vi "Controller - State Entry.vi"(8 "error in (no error)":errorcluster, 11 "View Model":T1) -> (0 "error out":errorcluster, 3 "View Model":T1)   [LabVIEW 2017]
doc: "Realized initial transition between current and next controller's states."
uses:
  Model/Controls/View Model.ctl
  Model/Controls/Shared Model.ctl
  Error Handler/Controls/Error Model.ctl
  Error Handler/Controls/Error Message.ctl
  Error Handler/Controls/Error Type.ctl
  Configuration/Controls/Config Model.ctl
  Configuration/Controls/Config DB Message.ctl
  Configuration/Controls/Config DB Command.ctl
  Configuration/Controls/Config DB Overhead.ctl
  Configuration/Controls/Config DB Record1.ctl
  Configuration/Controls/Config DB Record2.ctl
  Controls/Controller Wash Step.ctl
  Views/Vehicle Position Simulation View/Controls/Vehicle - Position.ctl
  Controls/Controller Model.ctl
  Controls/Controller Overhead.ctl
  Controls/Controller State.ctl
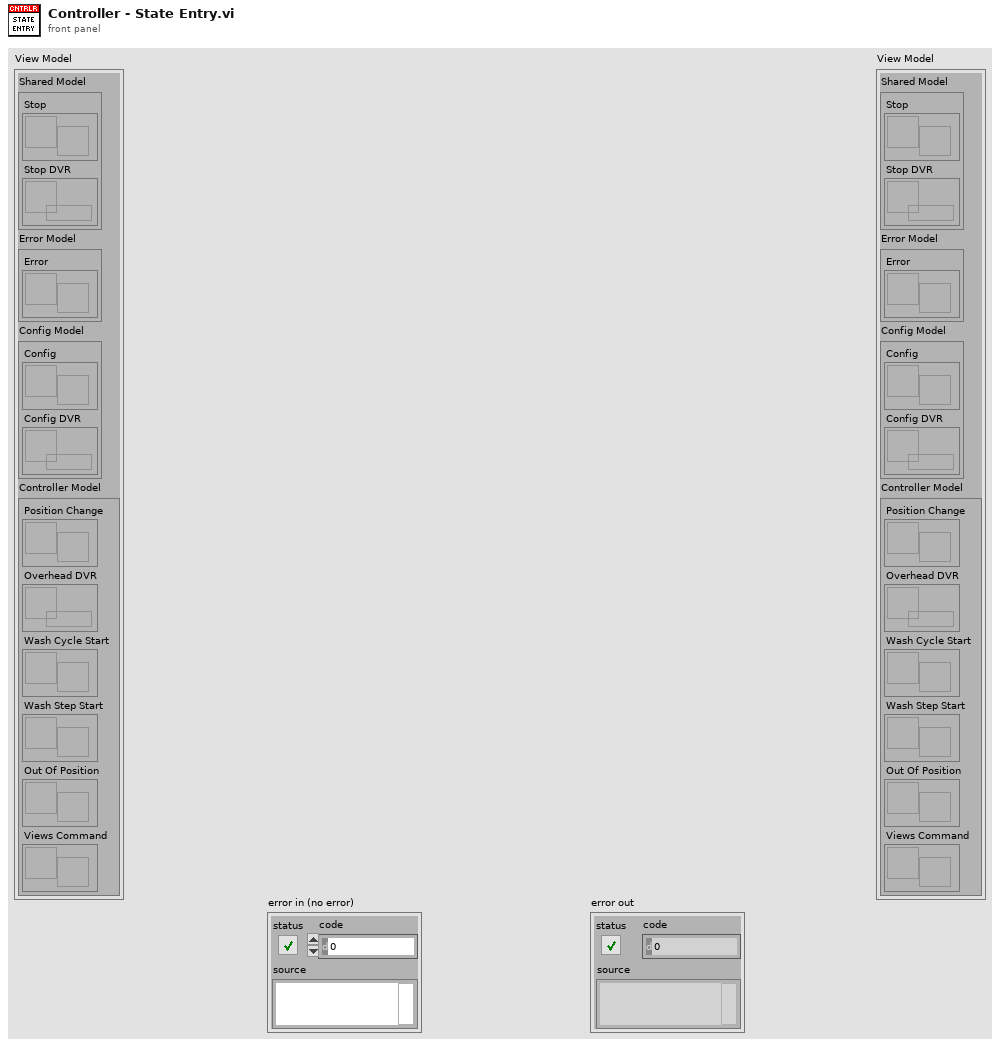
[diagram p1: front panel]
types:
  T1 = typedef "View Model.ctl" = cluster{"Shared Model":T2, "Error Model":T3, "Config Model":T4, "Controller Model":T5}
  T2 = typedef "Shared Model.ctl" = cluster{"Stop":refnum<user-event>, "Stop DVR":refnum<data-value>}
  T3 = typedef "Error Model.ctl" = cluster{"Error":refnum<user-event>}
  T4 = typedef "Config Model.ctl" = cluster{"Config":refnum<user-event>, "Config DVR":refnum<data-value>}
  T5 = typedef "Controller Model.ctl" = cluster{"Position Change":refnum<user-event>, "Overhead DVR":refnum<data-value>, "Wash Cycle Start":refnum<user-event>, "Wash Step Start":refnum<user-event>, "Out Of Position":refnum<user-event>, "Views Command":refnum<user-event>}
  T6 = typedef "Controller State.ctl" = enum16{"Initial", "Wait for Start", "Wash Cycle Start", "Wash Cycle Complete", "Wash Step Start", "Wash Step Execute", "Wash Step Complete", "Wait for Vehicle Position", "Wash Exit", "Wash Abort/Terminate"}
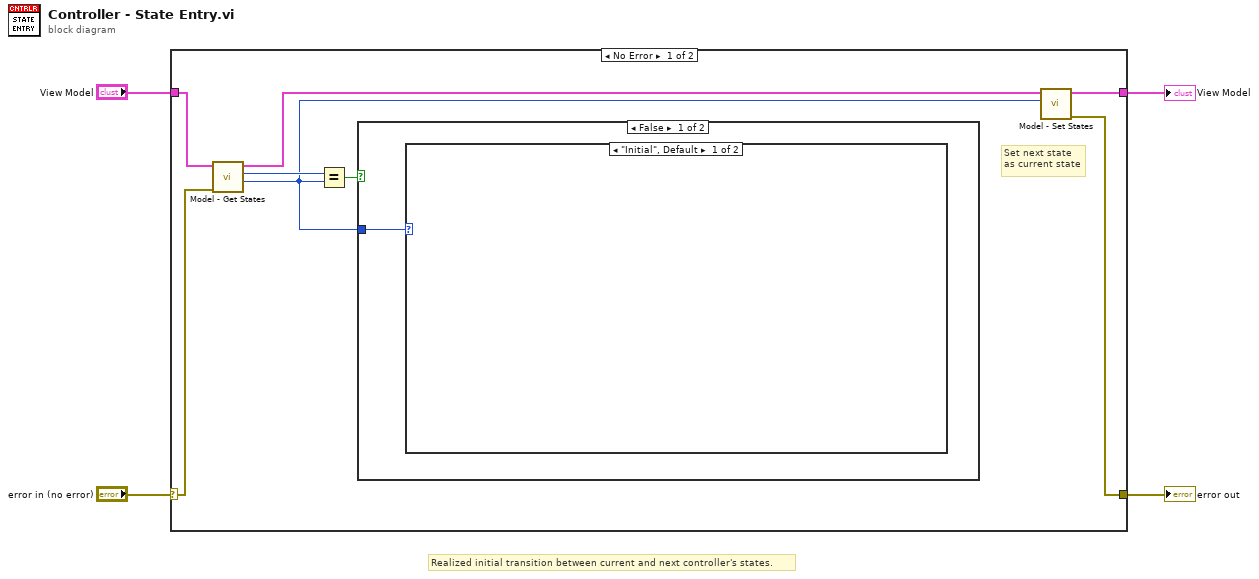
[diagram p0: block diagram]
diagram:
  # "Realized initial transition between current and next controller's states."
  n1 = case shown="No Error" "error in (no error)" {
    selector: "error in (no error)" -> [w11 w14]
    tunnel: "View Model" -> [w12 w15]
    tunnel: [w6 w14] -> w2
    tunnel: [w7 w15] -> w1
    frame No Error {
      # "Set next state\nas current state"
      n2 = call "Model - Get States.vi"("error in (no error)"=w11, "View Model"=w12) -> ("Next State"=w5:T6, "Current State"=w10:T6, "View Model"=w8:T1)  [unwired: 6 in, 1 out]
      n3 = Equal?(x=w10, y=w5) -> (x = y?=w9:bool)
      n4 = case shown="False" w9 {
        tunnel: w5 -> [w13 _]
        frame False {
          n5 = case shown="\"Initial\", Default" w13 {
            frame "Initial", Default {
            }
            frame "Wait for Start" {
            }
          }
        }
        frame True {
        }
      }
      n6 = call "Model - Set States.vi"("Current State"=w5, "View Model"=w8) -> ("error out"=w6:errorcluster, "View Model"=w7:T1)  [unwired: 8 in]
    }
    frame Error {
    }
  }
  "View Model" <- w1
  "error out" <- w2
